vi "ReadLabjackConfig(SubVI).vi"(8 "error in (no error)":errorcluster, 11 "appended path":path) -> (0 "error out":errorcluster, 3 "Utility":T1={"Ch1 Bias"="", "Ch2 Bias"="", "Ch3 Bias"="", "Ch4 Bias"="DAC0", "355 PWM"="", "AimingBeam PWM"="", "Laser Ready"="", "Interlock"="FIO1", "Laser Start/Stop"="FIO1", "Red LED"="FIO1", "Green LED"="DIO3", "Foot Pedal"="DIO15"})   [LabVIEW 2020]
uses:
  LJ Pin Setting.ctl
  <vilib>/Utility/file.llb/Read Delimited Spreadsheet (string).vi
  <vilib>/addons/_JKI.lib/Serialization/JSON/JKI JSON Serialization.lvlib
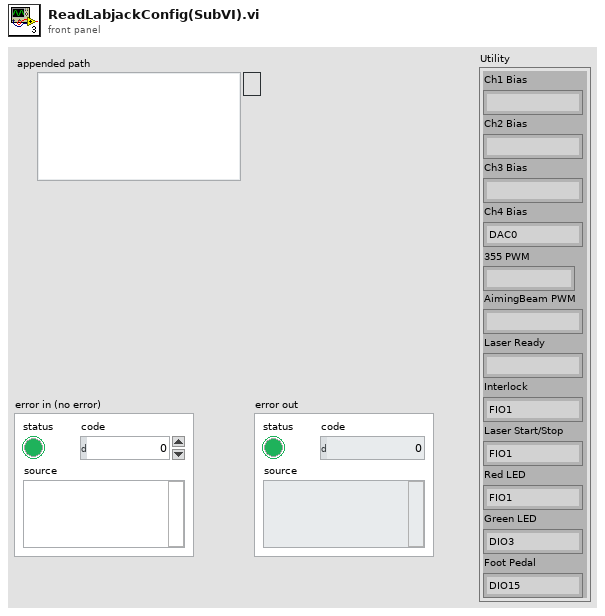
[diagram p1: front panel]
types:
  T1 = typedef "LJ Pin Setting.ctl" = cluster{"Ch1 Bias":string, "Ch2 Bias":string, "Ch3 Bias":string, "Ch4 Bias":string, "355 PWM":string, "AimingBeam PWM":string, "Laser Ready":string, "Interlock":string, "Laser Start/Stop":string, "Red LED":string, "Green LED":string, "Foot Pedal":string}
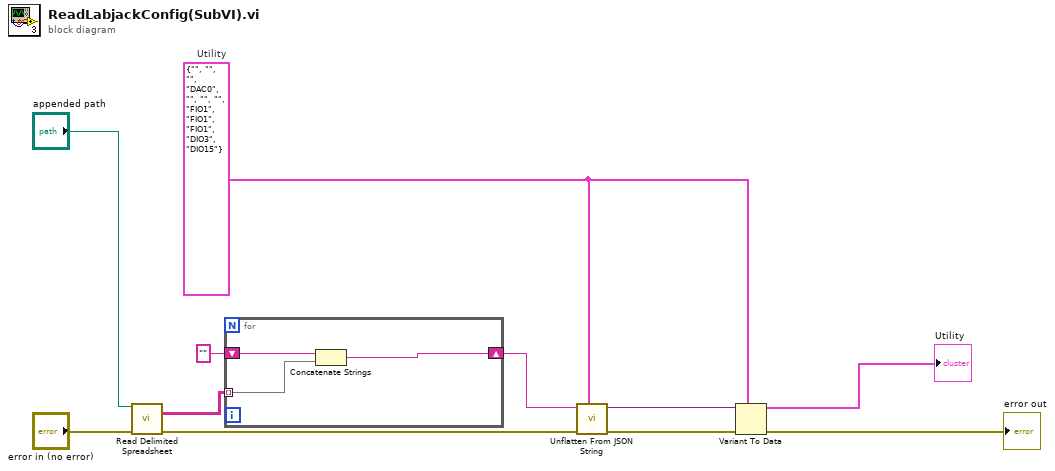
[diagram p0: block diagram]
diagram:
  w1 = T1 {"Ch1 Bias"="", "Ch2 Bias"="", "Ch3 Bias"="", "Ch4 Bias"="DAC0", "355 PWM"="", "AimingBeam PWM"="", "Laser Ready"="", "Interlock"="FIO1", "Laser Start/Stop"="FIO1", "Red LED"="FIO1", "Green LED"="DIO3", "Foot Pedal"="DIO15"}  # Utility
  n1 = call-poly <vilib>:"Read Delimited Spreadsheet.vi"("file path (dialog if empty)"="appended path", "error in (no error)"="error in (no error)") -> ("all rows"=w4:string[][], "error out"=w9:errorcluster)  [unwired: 8 in, 4 out]
  n2 = for {
    tunnel: w4 -> [w14] mode=indexing
    shift-right: [w12] -> w7
    shift-left: "" -> [w13]
    n3 = Concatenate Strings(w13, w14) -> (w12:string)
  }
  n4 = call <vilib>:"Unflatten From JSON String.vi"("Type and Defaults"=w1, "error in"=w9, "JSON String"=w7) -> ("error out"=w10:errorcluster, "Variant"=w6:variant)  [unwired: 7 in]
  n5 = Variant To Data(error in=w10, type=w1, Variant=w6) -> (data=→"Utility":T1, error out=→"error out":errorcluster)
